vi "Save Front Panel.vi"(8 "error in (no error)":errorcluster, 10 "path":path, 11 "vi ref":refnum<vi>) -> (0 "error out":errorcluster, 2 "path out":path, 3 "reference out":refnum<vi>)   [LabVIEW 2014, in "lvprj2html.lvlib"]
uses:
  lvprj2html.lvlib
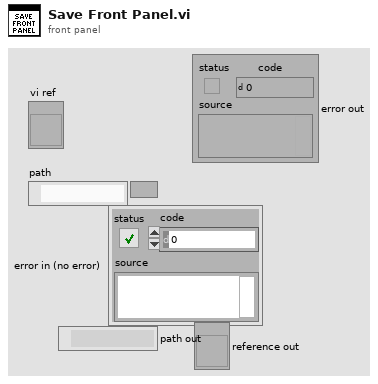
[diagram p1: front panel]
types:
  T1 = typedef "imagedata.ctl" = cluster{"image type":i32, "image depth":i32, "image":u8[], "mask":u8[], "colors":u32[], "Rectangle":cluster{"left":i16, "top":i16, "right":i16, "bottom":i16}}
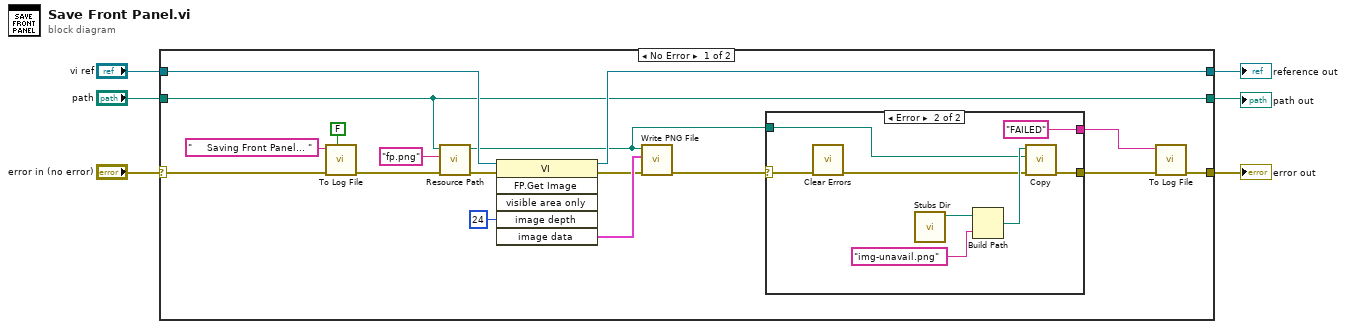
[diagram p0: block diagram]
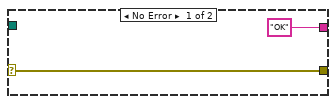
[diagram p2: hidden frame]
diagram:
  n1 = case shown="No Error" "error in (no error)" {
    selector: "error in (no error)" -> [w9 w34]
    tunnel: "vi ref" -> [w23 w35]
    tunnel: "path" -> [w13 w36]
    tunnel: [w17 w35] -> w4
    tunnel: [w14 w34] -> w3
    tunnel: [w13 w36] -> w1
    frame No Error {
      n2 = call "To Log File.vi"("new line"=FALSE, "error in (no error)"=w9, "string"="     Saving Front Panel... " ("format string")) -> ("error out"=w8:errorcluster)  [unwired: 8 in]
      n3 = call "Resource Path.vi"("error in (no error)"=w8, "resource file name"="fp.png", "data dir"=w13) -> ("error out"=w19:errorcluster, "path"=w7:path)  [unwired: 7 in]
      n4 = invoke class="VI" method="FP.Get Image"(reference=w23, error in=w19, "image depth"=24 ("Image Depth")) -> (reference out=w17:refnum<vi>, error out=w18:errorcluster, "image data"=w21:T1)  [unwired: 3 in, 3 out]
      n5 = call <vilib>:"Write PNG File.vi"("error in (no error)"=w18, "image data"=w21, "path to PNG file"=w7) -> ("error out"=w12:errorcluster)  [unwired: 7 in, 1 out]
      n6 = case shown="Error" w12 {
        selector: w12 -> [w25 w33]
        tunnel: [w25 w26] -> w10
        tunnel: ["OK" ("string") "FAILED" ("string")] -> w11
        tunnel: w7 -> [_ w28]
        frame No Error {
        }
        frame Error {
          n7 = call <vilib>:"Clear Errors.vi"("error in (no error)"=w33) -> ("error out"=w27:errorcluster)  [unwired: 5 in, 1 out]
          n8 = call "Stubs Dir.vi"() -> ("path"=w30:path)  [unwired: 11 in]
          n9 = Build Path(base path=w30, name or relative path="img-unavail.png") -> (appended path=w29:path)
          n10 = call "Copy.vi"("error in (no error)"=w27, "dst"=w28, "src"=w29) -> ("error out"=w26:errorcluster)  [unwired: 8 in]
        }
      }
      n11 = call "To Log File.vi"("error in (no error)"=w10, "string"=w11) -> ("error out"=w14:errorcluster)  [unwired: 9 in]
    }
    frame Error {
    }
  }
  "error out" <- w3
  "reference out" <- w4
  "path out" <- w1
